vi "setupPressureSensor.vi"(8 "error in (no error)":errorcluster, 10 "Model in":refnum<class "Model.lvclass">, 11 "Bootloader in":refnum<class "Bootloader.lvclass">) -> (0 "error out":errorcluster, 2 "Model out":refnum<class "Model.lvclass">, 3 "Bootloader out":refnum<class "Bootloader.lvclass">)   [LabVIEW 2015, in "Bootloader.lvclass"]
uses:
  Bootloader.lvclass
  Model/Model.lvclass
  PressureSensor/PressureSensor/PressureSensor.lvclass
  Typedefs/Pressure Sensor Settings.ctl
  Model/Model.lvclass/Model.ctl
  ConfigurationTestParameters/ConfigurationTestParameters.lvclass
  Typedefs/FAMTTypedefs.lvlib
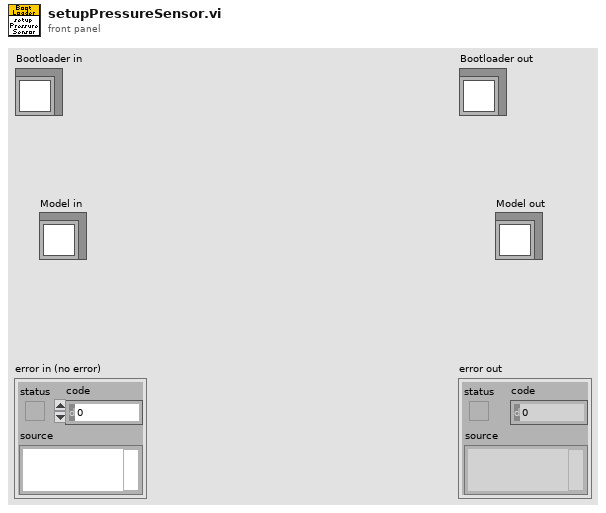
[diagram p1: front panel]
types:
  T1 = typedef "FAMTTypedefs.lvlib/Pressure Sensor Settings.ctl" = cluster{"Channel":tag, "Terminal Configuration":i32, "Minimum":dbl[unit], "Maximum":dbl[unit]}
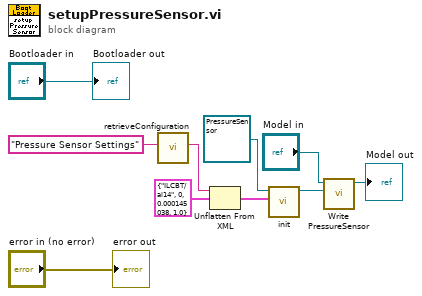
[diagram p0: block diagram]
diagram:
  n1 = call "retrieveConfiguration.vi"("configName"="Pressure Sensor Settings") -> ("xmlConfig"=w2:string)  [unwired: 8 in, 2 out]
  n2 = Unflatten From XML(xml string=w2, type=T1 {"Channel"="ILCBT/ai14", "Terminal Configuration"=0, "Minimum"=0.000145038, "Maximum"=1.0} ("Pressure Sensor Settings")) -> (value=w1:T1)  [unwired: 1 in, 1 out]
  n3 = call "init.vi"("Pressure Sensor Settings"=w1, "PressureSensor in"=refnum<class "PressureSensor.lvclass"> refnum ("PressureSensor.lvclass")) -> ("PressureSensor out"=w7:refnum<class "PressureSensor.lvclass">)  [unwired: 8 in, 1 out]
  n4 = call "Write PressureSensor.vi"("PressureSensor"=w7, "Model in"="Model in") -> ("Model out"=→"Model out":refnum<class "Model.lvclass">)  [unwired: 9 in]
  "error out" <- "error in (no error)"
  "Bootloader out" <- "Bootloader in"
